vi "cameras_test.vi"() -> ()   [LabVIEW 2023]
doc: "Use this template to build a user interface event handler design pattern. Use this pattern for dialog boxes and other user interfaces. You also can create and execute user-defined events that the VI can handle the same way as user interface events."
uses:
  camera.ctl
  camera driver.ctl
  Vision.lvlib
panel:
  in  "Enable imaqdx":bool
  out "String":string
  in  "info tabs":enum32{"Modes", "Properties"}(tab)
  out "Available modes":string
  out "properties":string
  out "Image":T1(plugin-control)
  in  "Save Config":bool
  in  "Open Camera":bool
  out "Camera Selection":T2[](array[typedef])
  in  "stop":bool
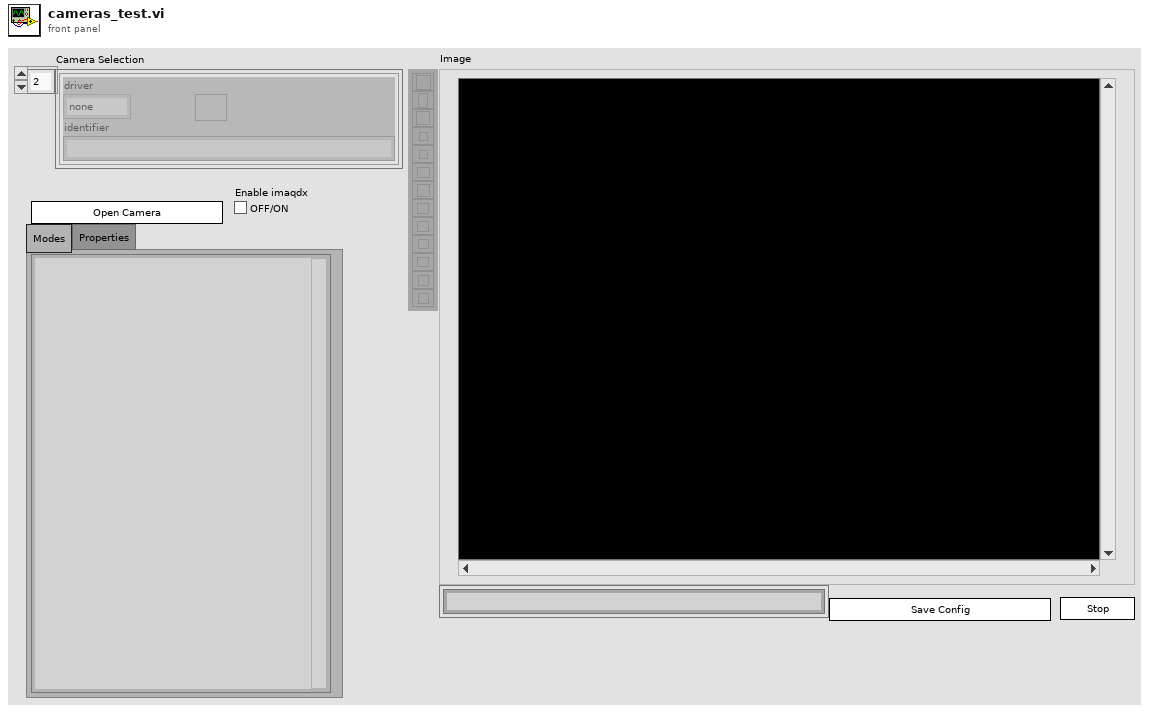
[diagram p1: front panel]
types:
  T1 = typedef "IMAQ Image.ctl" = refnum<image>
  T2 = typedef "Vision.lvlib/camera.ctl" = cluster{"camera reference":variant, "driver":T3, "identifier":string}
  T3 = typedef "Vision.lvlib/camera driver.ctl" = enum16{"none", "ueye", "wmf", "imaqdx"}
  T4 = typedef "camera mode.ctl" = cluster{"id":i32, "width":i32, "height":i32, "framerate":sgl}
  T5 = cluster{"prop name":string, "value":sgl, "auto":bool}[]
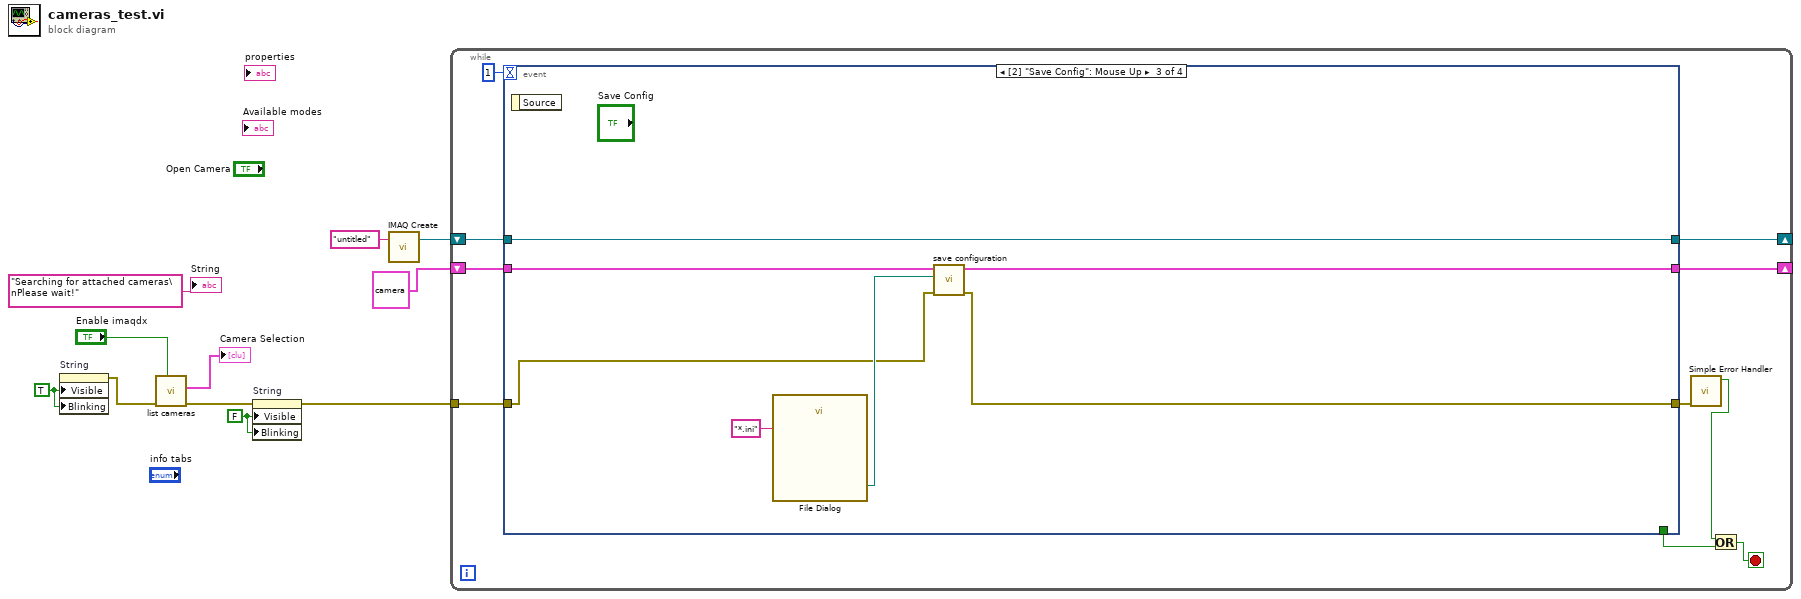
[diagram p0: block diagram]
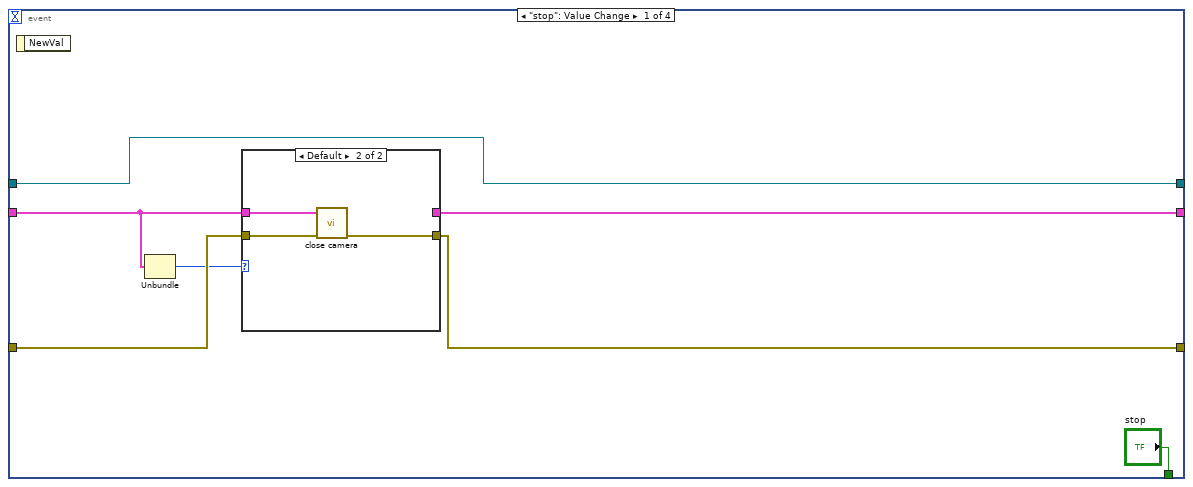
[diagram p2: hidden frame]
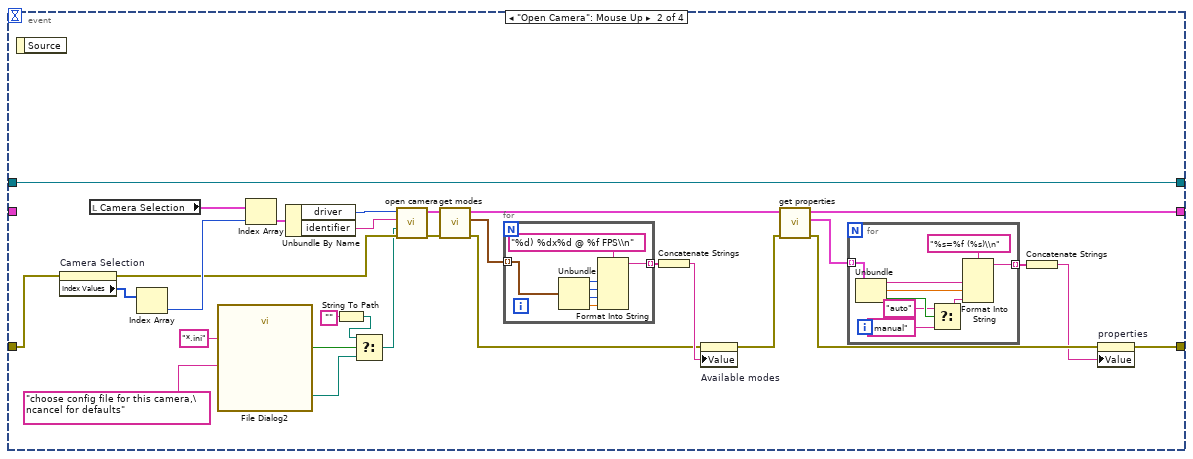
[diagram p4: hidden frame]
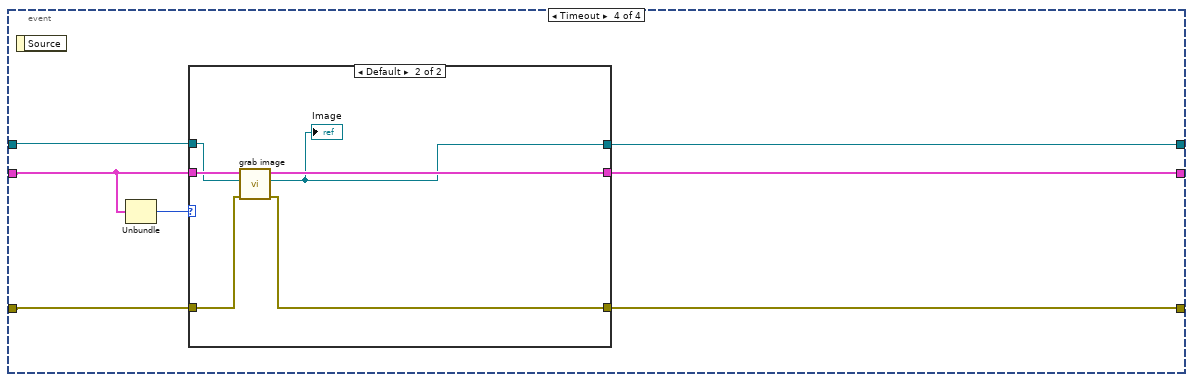
[diagram p5: hidden frame]
diagram:
  w3 = FALSE ("Visible")
  w5 = TRUE ("Visible")
  n1 = property on="String" class="Str"("Visible"=w5, "Blinking"=w5) -> (error out=w6:errorcluster)  [unwired: 2 in, 1 out]
  n2 = call "list cameras.vi"("Enable imaqdx"="Enable imaqdx", "error in (no error)"=w6) -> ("error out"=w4:errorcluster, "Cameras"=→"Camera Selection":T2[])  [unwired: 8 in]
  n3 = property on="String" class="Str"(error in=w4, "Visible"=w3, "Blinking"=w3) -> (error out=w2:errorcluster)  [unwired: 1 in, 1 out]
  n4 = call "IMAQ Create"("Image Name"="untitled") -> ("New Image"=w10:T1)  [unwired: 4 in, 1 out]
  n5 = while {
    tunnel: w2 -> [w19]
    shift-right: [w17] -> _
    shift-left: T2 {"camera reference"=variant, "driver"=enum."none", "identifier"=""} ("Camera") -> [w16]
    shift-right: [w15] -> _
    shift-left: w10 -> [w20]
    stop <- w12 stop-if-true
    n6 = event shown="[2] \"Save Config\": Mouse Up" {
      selector: _ -> [_ _ _ _]
      dyn-events: _ -> [_ _ _ _]
      timeout: 1 -> [_ _ _ _]
      tunnel: ["stop" _ _ _] -> w14
      tunnel: w20 -> [w22 w53 w84 w91]
      tunnel: w19 -> [w27 w59 w82 w90]
      tunnel: [w23 w41 w83 w89] -> w18
      tunnel: [w22 w53 w84 w87] -> w15
      tunnel: [w24 w44 w81 w88] -> w17
      tunnel: w16 -> [w26 _ w80 w92]
      event "stop": Value Change {
        n7 = event-data() -> ()  [unwired: 1 in, 1 out]
        n8 = Unbundle(w26) -> ("driver"=w25:T3)  [unwired: 2 out]
        n9 = case shown="Default" w25 {
          tunnel: w26 -> [w30 w33]
          tunnel: w27 -> [w29 w32]
          tunnel: [w30 _] -> w24
          tunnel: [w29 w31] -> w23
          frame "none" {
          }
          frame Default {
            n10 = call "close camera.vi"("error in (no error)"=w32, "Camera"=w33) -> ("error out"=w31:errorcluster)  [unwired: 8 in, 1 out]
          }
        }
      }
      event "Open Camera": Mouse Up {
        n11 = event-data() -> ()  [unwired: 1 in, 1 out]
        n12 = property on="Camera Selection" class="Arr (strict)"(error in=w59) -> (error out=w56:errorcluster, "Index Values"=w60:u32[])  [unwired: 1 in, 1 out]
        n13 = local read "Camera Selection"() -> (w57:T2[])
        n14 = Index Array(array=w60) -> (element=w58:u32)  [unwired: 1 in]
        n15 = call "File Dialog2"("prompt"="choose config file for this camera,\ncancel for defaults", "pattern (all files)"="*.ini") -> ("selected path"=w37:path, "cancelled"=w38:bool)  [unwired: 10 in, 2 out]
        n16 = Index Array(array=w57, index=w58) -> (element=w63:T2)
        n17 = Unbundle By Name(w63) -> ("driver"=w61:T3, "identifier"=w62:string)
        n18 = String To Path(string="") -> (path=w35:path)
        n19 = Select(t=w35, s=w38, f=w37) -> (s? t:f=w36:path)
        n20 = call "open camera.vi"("error in (no error)"=w56, "Camera Settings"=w36, "identifier"=w62, "driver"=w61) -> ("error out"=w51:errorcluster, "Camera"=w52:T2)  [unwired: 6 in]
        n21 = call "get modes.vi"("error in (no error)"=w51, "Camera"=w52) -> ("error out"=w47:errorcluster, "Modes"=w50:T4[], "Camera out"=w46:T2)  [unwired: 7 in]
        n22 = for {
          tunnel: w50 -> [w78] mode=indexing
          tunnel: [w73] -> w49 mode=indexing
          n23 = Unbundle(w78) -> ("id"=w77:i32, "width"=w76:i32, "height"=w75:i32, "framerate"=w74:sgl)
          n24 = Format Into String(format string="%d) %dx%d @ %f FPS\\n", w77, w76, w75, w74) -> (resulting string=w73:string)  [unwired: 2 in, 1 out]
        }
        n25 = Concatenate Strings(w49) -> (w48:string)
        n26 = property on="Available modes" class="Str"(error in=w47, "Value"=w48) -> (error out=w45:errorcluster)  [unwired: 1 in, 1 out]
        n27 = call "get properties.vi"("error in (no error)"=w45, "Camera"=w46) -> ("error out"=w42:errorcluster, "Properties"=w43:T5, "Camera out"=w44:T2)  [unwired: 7 in]
        n28 = for {
          tunnel: w43 -> [w71] mode=indexing
          tunnel: [w69] -> w40 mode=indexing
          n29 = Unbundle(w71) -> ("prop name"=w68:string, "value"=w70:sgl, "auto"=w67:bool)
          n30 = Select(t="auto", s=w67, f="manual") -> (s? t:f=w64:string)
          n31 = Format Into String(format string="%s=%f (%s)\\n", w68, w70, w64) -> (resulting string=w69:string)  [unwired: 2 in, 1 out]
        }
        n32 = Concatenate Strings(w40) -> (w39:string)
        n33 = property on="properties" class="Str"(error in=w42, "Value"=w39) -> (error out=w41:errorcluster)  [unwired: 1 in, 1 out]
      }
      event "Save Config": Mouse Up {
        n34 = event-data() -> ()  [unwired: 1 in, 1 out]
        n35 = call "File Dialog"("pattern (all files)"="*.ini" ("pattern label")) -> ("selected path"=w86:path)  [unwired: 11 in, 3 out]
        n36 = call "save configuration.vi"("error in (no error)"=w82, "Path"=w86, "Camera"=w80) -> ("error out"=w83:errorcluster, "Camera out"=w81:T2)  [unwired: 7 in]
      }
      event Timeout {
        n37 = event-data() -> ()  [unwired: 1 in, 1 out]
        n38 = Unbundle(w92) -> ("driver"=w93:T3)  [unwired: 2 out]
        n39 = case shown="Default" w93 {
          tunnel: w92 -> [w94 w102]
          tunnel: w91 -> [w96 w101]
          tunnel: [w94 w100] -> w88
          tunnel: w90 -> [w95 w99]
          tunnel: [w95 w98] -> w89
          tunnel: [w96 w97] -> w87
          frame "none" {
          }
          frame Default {
            n40 = call "grab image.vi"("error in (no error)"=w99, "Image In"=w101, "Camera"=w102) -> ("error out"=w98:errorcluster, "Image Out"=w97:T1, "Camera out"=w100:T2)  [unwired: 6 in]
            "Image" <- w97
          }
        }
      }
    }
    n41 = call <vilib>:"Simple Error Handler.vi"("error in (no error)"=w18) -> ("error?"=w13:bool)  [unwired: 4 in, 4 out]
    n42 = Or(x=w13, y=w14) -> (x .or. y?=w12:bool)
  }
  "String" <- "Searching for attached cameras\nPlease wait!" ("String")
